vi "Read useTerminate.vi"(8 "error in (no error)":errorcluster, 11 "MotorControllerClass in":refnum<class "MotorControllerClass.lvclass">) -> (0 "error out":errorcluster, 2 "useTerminate":bool, 3 "MotorControllerClass out":refnum<class "MotorControllerClass.lvclass">)   [LabVIEW 2018, in "MotorControllerClass.lvclass"]
uses:
  BMS/MotorControllerClass.lvclass
  BMS/MotorControllerClass.lvclass/MotorControllerClass.ctl
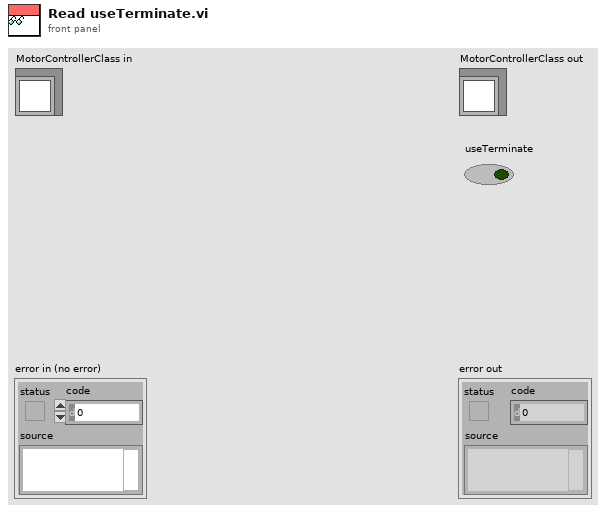
[diagram p1: front panel]
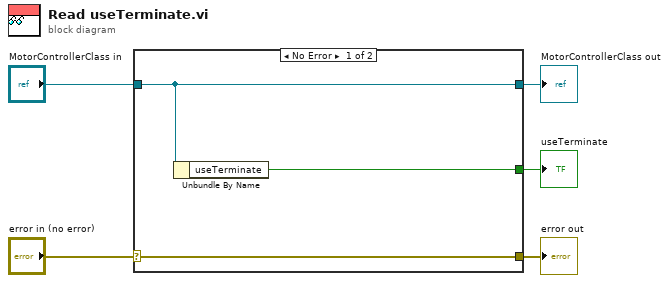
[diagram p0: block diagram]
diagram:
  n1 = case shown="No Error" "error in (no error)" {
    selector: "error in (no error)" -> [w8 w9]
    tunnel: [w8 w9] -> w4
    tunnel: [w7 w10] -> w2
    tunnel: "MotorControllerClass in" -> [w7 w10]
    tunnel: [w6 _] -> w1
    frame No Error {
      n2 = Unbundle By Name(w7) -> ("useTerminate"=w6:bool)
    }
    frame Error {
    }
  }
  "error out" <- w4
  "MotorControllerClass out" <- w2
  "useTerminate" <- w1
